vi "timestamp to file compatible string.vi"(6 "time stamp":timestamp, 8 "error constant":errorcluster) -> (0 "error IO":errorcluster, 4 "date/time string":string)   [LabVIEW 2012]
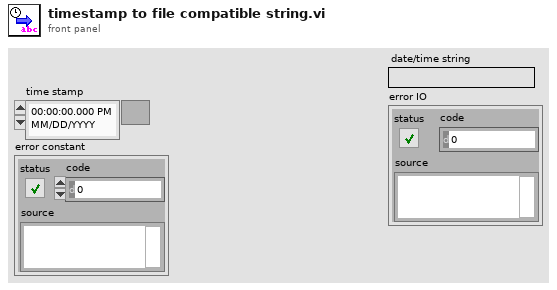
[diagram p1: front panel]
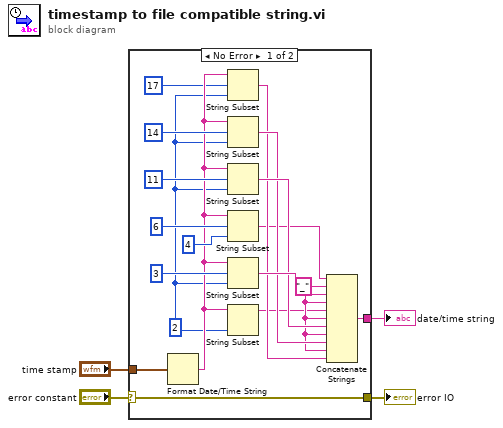
[diagram p0: block diagram]
diagram:
  n1 = case shown="No Error" "error constant" {
    selector: "error constant" -> [w5 w23]
    tunnel: [w17 _] -> w4
    tunnel: "time stamp" -> [w6 _]
    tunnel: [w5 w23] -> w1
    frame No Error {
      w7 = 2 ("length (rest)")
      w11 = "_" ("string")
      n2 = Format Date/Time String(seconds (now)=w6) -> (date/time string=w13:string)  [unwired: 2 in]
      n3 = String Subset(string=w13, offset (0)=17, length (rest)=w7) -> (substring=w10:string)
      n4 = String Subset(string=w13, offset (0)=14, length (rest)=w7) -> (substring=w14:string)
      n5 = String Subset(string=w13, offset (0)=11, length (rest)=w7) -> (substring=w19:string)
      n6 = String Subset(string=w13, offset (0)=6, length (rest)=4 ("length (rest)")) -> (substring=w9:string)
      n7 = String Subset(string=w13, offset (0)=3, length (rest)=w7) -> (substring=w21:string)
      n8 = String Subset(string=w13, length (rest)=w7) -> (substring=w8:string)  [unwired: 1 in]
      n9 = Concatenate Strings(w9, w11, w21, w11, w8, w11, w19, w11, w14, w11, w10) -> (w17:string)
    }
    frame Error {
    }
  }
  "date/time string" <- w4
  "error IO" <- w1
